vi "Generation of Square wave from sine waves.vi"() -> ()   [LabVIEW 2009]
uses:
  <vilib>/Analysis/NI_AALBase.lvlib
panel:
  out "Individual sines":dbl[][](graph)
  in  "stop":bool
  in  "# of Sines":i32(slide) step=1 scale=0.0..50.0
  out "Sum of Sines":dbl[](graph)
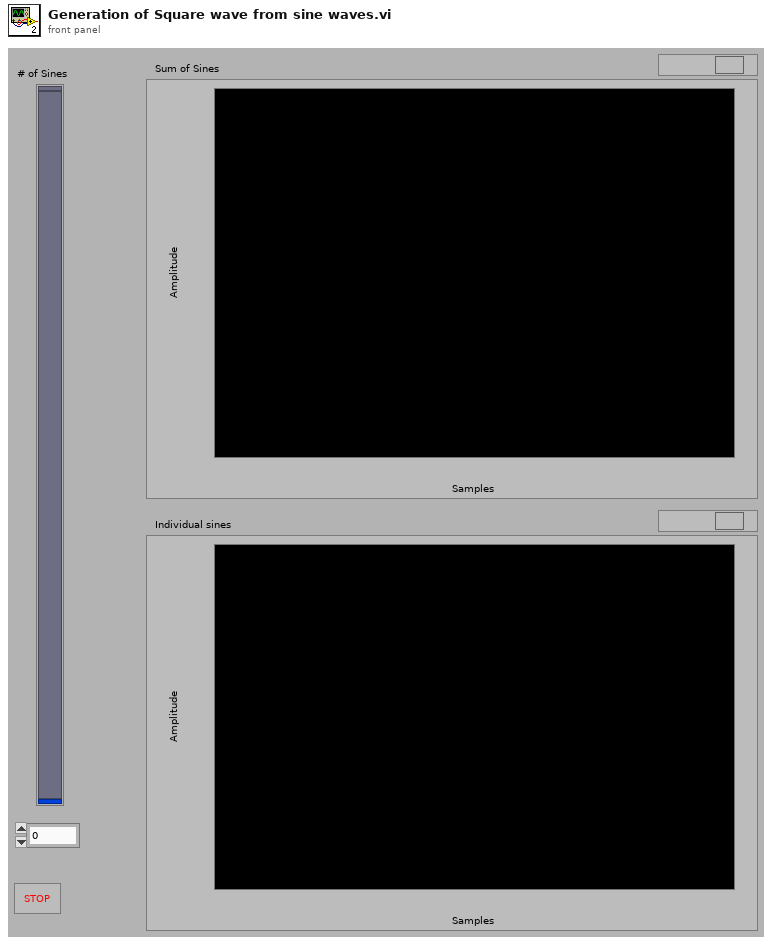
[diagram p1: front panel]
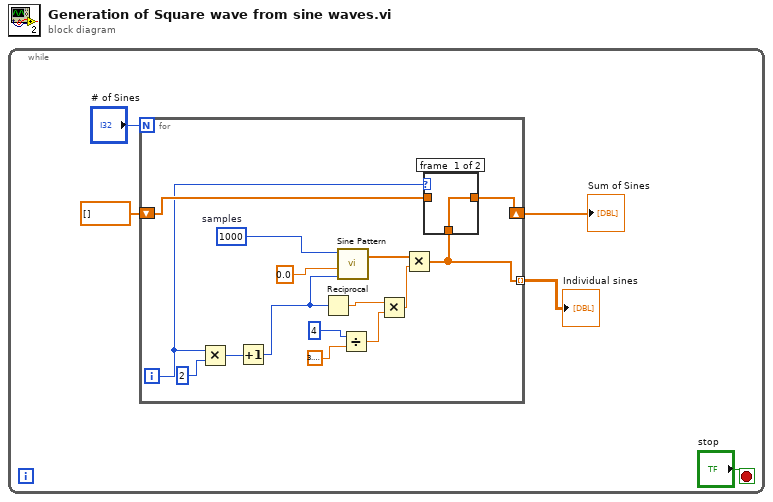
[diagram p0: block diagram]
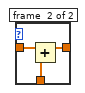
[diagram p2: hidden frame]
diagram:
  n1 = while {
    stop <- "stop" stop-if-true
    n2 = for {
      N: "# of Sines" -> [_]
      shift-right: [w18] -> w5
      shift-left: dbl[] [] ("Sinusoidal Pattern") -> [w19]
      tunnel: [w6] -> w1 mode=indexing
      i -> [w17]
      w20 = 1000  # samples
      n3 = Multiply(x=w17, y=2) -> (x*y=w15:i32)
      n4 = Increment(x=w15) -> (x+1=w14:i32)
      n5 = Reciprocal(x=w14) -> (1/x=w8:dbl)
      n6 = call <vilib>:"Sine Pattern.vi"("cycles"=w14, "phase(degrees)"=0.0, "samples"=w20) -> ("Sinusoidal Pattern"=w13:dbl[])  [unwired: 1 in, 1 out]
      n7 = Divide(x=4 ("y"), y=3.141592653589793) -> (x/y=w9:dbl)
      n8 = Multiply(x=w8, y=w9) -> (x*y=w7:dbl)
      n9 = Multiply(x=w13, y=w7) -> (x*y=w6:dbl[])
      n10 = case shown="Default" w17 {
        tunnel: [w21 w24] -> w18
        tunnel: w19 -> [_ w23]
        tunnel: w6 -> [w21 w22]
        frame #0 {
        }
        frame #1 {
          n11 = Add(x=w23, y=w22) -> (x+y=w24:dbl[])
        }
      }
    }
    "Sum of Sines" <- w5
    "Individual sines" <- w1
  }
